vi "Buffer.vi"(4 "Function":enum16{"Read", "Insert"}(ring), 5 "Error In":errorcluster, 7 "Plugin Name":T1, 8 "Reference In":refnum<vi>) -> (0 "Error Out":errorcluster, 3 "Reference Out":refnum<vi>)   [LabVIEW 2015, in "Plugin Chart References.lvlib"]
uses:
  Plugin Chart References.lvlib
  _libraries/Startup Processes/_typedefs/Subpanel Names.ctl
  _libraries/Startup Processes/Startup Processes.lvlib
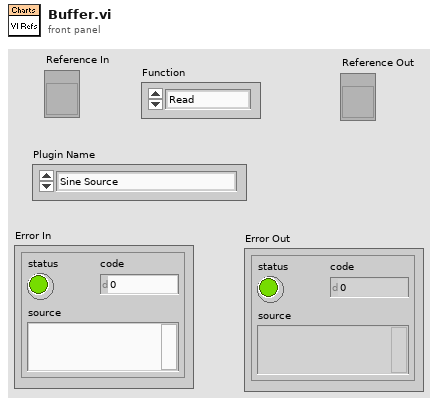
[diagram p1: front panel]
types:
  T1 = typedef "Startup Processes.lvlib/Subpanel Names.ctl" = enum16{"Sine Source", "Ramp Source", "Hen House TC", "Dog House TC", "Out House TC"}
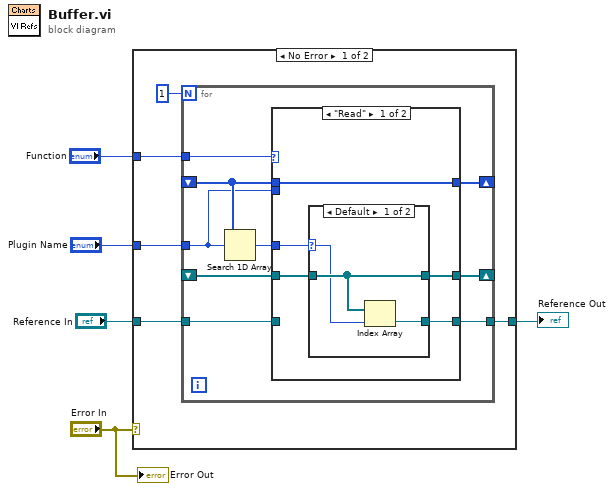
[diagram p0: block diagram]
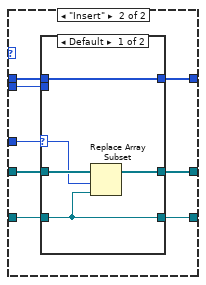
[diagram p3: hidden frame]
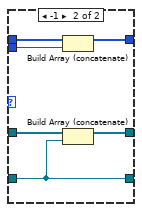
[diagram p4: hidden frame]
diagram:
  n1 = case shown="No Error" "Error In" {
    tunnel: "Function" -> [w9 _]
    tunnel: "Reference In" -> [w8 _]
    tunnel: [w7 _] -> w2
    tunnel: "Plugin Name" -> [w6 _]
    frame No Error {
      n2 = for {
        N: 1 -> [_]
        tunnel: w9 -> [w19]
        shift-right: [w17] -> _
        shift-left: _ -> [w18]
        tunnel: w8 -> [w16]
        tunnel: [w15] -> w7
        shift-right: [w13] -> _
        shift-left: _ -> [w14]
        tunnel: w6 -> [w12]
        n3 = Search 1D Array(1D array=w14, element=w12) -> (index of element=w11:i32)  [unwired: 1 in]
        n4 = case shown="\"Read\"" w19 {
          tunnel: w18 -> [w24 w36]
          tunnel: [w22 w35] -> w17
          tunnel: w16 -> [_ w34]
          tunnel: [w21 w30] -> w15
          tunnel: w14 -> [w20 w33]
          tunnel: [w20 w32] -> w13
          tunnel: w12 -> [_ w31]
          tunnel: w11 -> [w23 w29]
          frame "Read" {
            n5 = case shown="Default" w23 {
              selector: w23 -> [w25 _]
              tunnel: w24 -> [w26 w28]
              tunnel: [w26 w28] -> w22
              tunnel: [w27 _] -> w21
              frame Default {
                n6 = Index Array(array=w26, index=w25) -> (element=w27:refnum<vi>)
              }
              frame -1 {
              }
            }
          }
          frame "Insert" {
            n7 = case shown="Default" w29 {
              selector: w29 -> [w37 _]
              tunnel: w36 -> [w40 w47]
              tunnel: [w39 w46] -> w35
              tunnel: w34 -> [w38 w42]
              tunnel: w33 -> [w41 w45]
              tunnel: [w41 w44] -> w32
              tunnel: w31 -> [_ w43]
              tunnel: [w38 w42] -> w30
              frame Default {
                n8 = Replace Array Subset(array=w40, new element=w38, index=w37) -> (w39:refnum<vi>[])
              }
              frame -1 {
                n9 = Build Array (concatenate)(w45, w43) -> (w44:T1[])
                n10 = Build Array (concatenate)(w47, w42) -> (w46:refnum<vi>[])
              }
            }
          }
        }
      }
    }
    frame Error {
    }
  }
  "Reference Out" <- w2
  "Error Out" <- "Error In"
